vi "KP_KI_Integration2.vi"() -> ()   [LabVIEW 2023]
panel:
  in  "ip":cdb[][][][][][][][][][][][][][][][][][][](array[numeric])
  in  "op":cdb[][][][][][][][][][][][][][][][][][][](array[numeric])
  out "Ki":dbl
  out "Kp":dbl
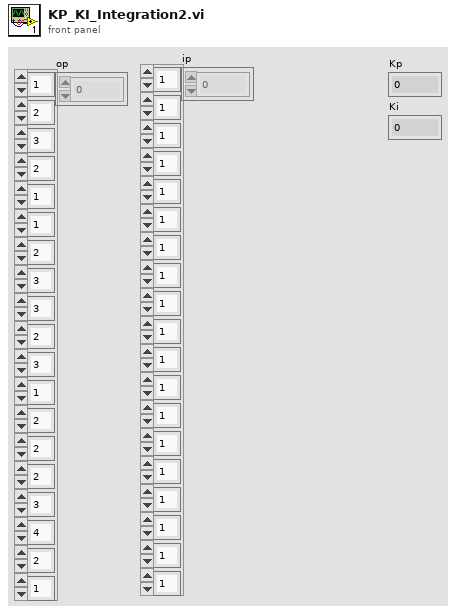
[diagram p1: front panel]
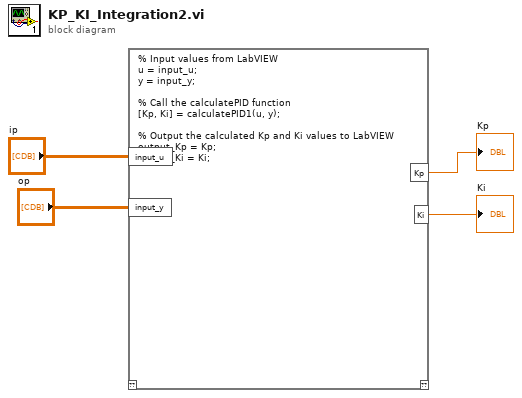
[diagram p0: block diagram]
diagram:
  n1 = script code="% Input values from LabVIEW\nu = input_u;\ny = input_y;\n\n% Call the calculatePID function\n[Kp, Ki] = calculatePID1(u, y);\n\n% Output the calculated Kp and Ki values to LabVIEW\noutput_Kp = Kp;\noutput_Ki = Ki;"("input_u"="ip", "input_y"="op") -> ("Kp"=→"Kp":dbl, "Ki"=→"Ki":dbl)  [unwired: 1 in, 1 out]
